vi "Gui_SetupExpert.vi"(8 "error in (no error)":errorcluster, 11 "QMH UI References.Refnum EXPERT":refnum<vi>) -> (0 "error out":errorcluster caption="sortie d'erreur")   [LabVIEW 2024]
doc: "This VI setup the EXPERT parameters.\n\n1. The EXPERT parameters are passed through a Reference as input.\n2. Init the controls with the previous values.\n3. Wait for the user events, and update controls accordingly.\n4. When OK is pushed, the last values of the controls are stored into the address passed by Reference."
uses:
  controls/EXPERT_Inputs.ctl
  controls/DIGIT_5122_Inputs.ctl
  <instrlib>/niScope/Controls/niScope trigger source.ctl
  controls/HSDIO_6541_Inputs.ctl
  <instrlib>/niHSDIO/niHSDIO.llb/niHSDIO_ctl Trigger Source Values (Ring).ctl
  controls/SOFTWARE_Inputs.ctl
  controls/AO_6711_Inputs.ctl
  controls/AWG_5421_Inputs.ctl
  <instrlib>/niFgen/niFgen.llb/niFgen_ctl Trigger Source Values (Ring).ctl
  controls/XML_Inputs.ctl
  controls/AO_6738_Inputs.ctl
panel:
  in  "EXPERT Inputs":T1={"XML Inputs"={"Version Tag Name"="XML_Version", "Version String"="1.0"}, "SOFTWARE Inputs"={"Application Directory"=path "D:/S.O.F.T.S/LABVIEW/PIL", "Software Version"="1.0.0", "Data Path"=path "D:/PIRENEA/DATA", "XML Path"=path "D:/PIRENEA/DATA", "XML File Filter"="*.xml", "XML Saved Path"=path "D:/PIRENEA/DATA/SAVED", "Excit Scripts Path"=path "D:/PIRENEA/EXCIT_SCRIPTS", "Excit Scripts File Filter"="*.txt", "Excit Waveforms Path"=path "D:/PIRENEA/EXCIT_WFMS", "Excit Waveforms File Filter"="*.bin", "Timing Scripts Path"=path "D:/PIRENEA/TIMING_SCRIPTS", "Timing Scripts File Filter"="*.txt", "Timing Waveforms Path"=path "D:/PIRENEA/TIMING_WFMS", "Timing Waveforms File Filter"="*.bin", "Trapping Waveforms Path"=path "D:/PIRENEA/TRAPPING_WFMS", "Trapping Waveforms File Filter"="*.bin"}, "HSDIO 6541 Inputs"={"Resource Name"="HSDIO_6541", "Clock Rate"=1000000.0, "Trigger Source"="PFI0"}, "AWG 5421 Inputs"={"Resource Name"="AWG_5421", "Sample Rate"=10000000.0, "Trigger Type"=2, "Trigger Source"="PFI0", "Waveform Gain"=0.31, "Digital Filter ON"=TRUE}, "DIGIT 5122 Inputs"={"Sample Rate"=10000.0, "Resource Name"="DIGIT_5122", "Channel Name"="0", "Trigger Source"="VAL_EXTERNAL", "Vertical Range"=10.0, "Trigger Level"=3.0}, "AO 6711 Inputs"={"Physical Channels"="AO_6711/ao0:3", "Min Voltage"=-10.0, "Max Voltage"=10.0, "Trigger Source"="/AO_6711/PFI3", "Counter"="AO_6711/ctr0"}, "AO 6738 Inputs"={"Physical Channels"="AO_6738/ao0:3", "Min Voltage"=-10.0, "Max Voltage"=10.0, "Trigger Source"="/AO_6738/PFI2", "Counter"="AO_6738/ctr0"}} {"AO 6738 Inputs"."Max Voltage" min=-10.0 max=10.0; "AO 6738 Inputs"."Min Voltage" min=-10.0 max=10.0; "AWG 5421 Inputs"."Sample Rate" format="%.2p"; "AWG 5421 Inputs"."Trigger Type" items=["None", "Software Edge", "Digital Edge", "Digital Level"]; "AO 6711 Inputs"."Max Voltage" min=-10.0 max=10.0; "AO 6711 Inputs"."Min Voltage" min=-10.0 max=10.0; "HSDIO 6541 Inputs"."Clock Rate" format="%.2p"; "DIGIT 5122 Inputs"."Trigger Level" format="%.2f"; "DIGIT 5122 Inputs"."Vertical Range" format="%.2f"; "DIGIT 5122 Inputs"."Sample Rate" step=65535.0 format="%#_3p"}
  in  "OK":bool
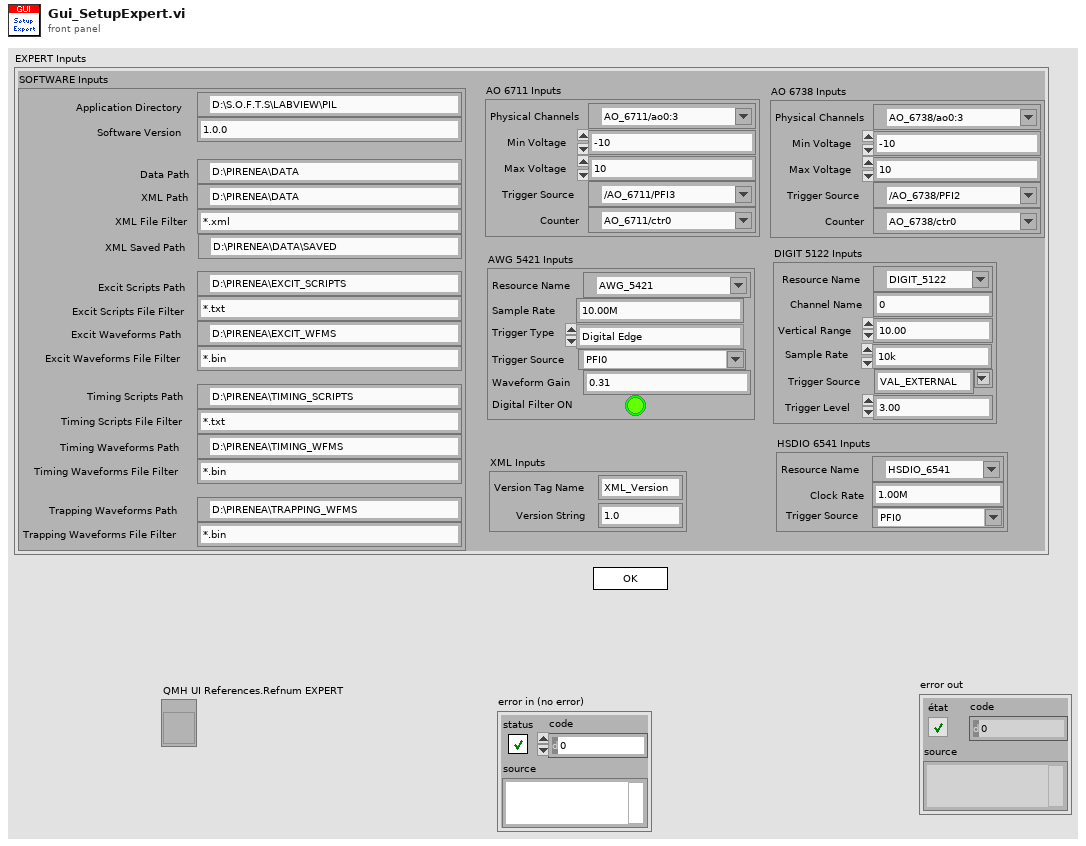
[diagram p1: front panel]
types:
  T1 = typedef "EXPERT_Inputs.ctl" = cluster{"XML Inputs":T2, "SOFTWARE Inputs":T3, "HSDIO 6541 Inputs":T4, "AWG 5421 Inputs":T6, "DIGIT 5122 Inputs":T8, "AO 6711 Inputs":T10, "AO 6738 Inputs":T11}
  T2 = typedef "XML_Inputs.ctl" = cluster{"Version Tag Name":string, "Version String":string}
  T3 = typedef "SOFTWARE_Inputs.ctl" = cluster{"Application Directory":path, "Software Version":string, "Data Path":path, "XML Path":path, "XML File Filter":string, "XML Saved Path":path, "Excit Scripts Path":path, "Excit Scripts File Filter":string, "Excit Waveforms Path":path, "Excit Waveforms File Filter":string, "Timing Scripts Path":path, "Timing Scripts File Filter":string, "Timing Waveforms Path":path, "Timing Waveforms File Filter":string, "Trapping Waveforms Path":path, "Trapping Waveforms File Filter":string}
  T4 = typedef "HSDIO_6541_Inputs.ctl" = cluster{"Resource Name":refnum<k15>, "Clock Rate":dbl, "Trigger Source":T5}
  T5 = typedef "niHSDIO_ctl Trigger Source Values (Ring).ctl" = string
  T6 = typedef "AWG_5421_Inputs.ctl" = cluster{"Resource Name":refnum<k15>, "Sample Rate":dbl, "Trigger Type":u16, "Trigger Source":T7, "Waveform Gain":dbl, "Digital Filter ON":bool}
  T7 = typedef "niFgen_ctl Trigger Source Values (Ring).ctl" = string
  T8 = typedef "DIGIT_5122_Inputs.ctl" = cluster{"Sample Rate":dbl, "Resource Name":refnum<k15>, "Channel Name":string, "Trigger Source":T9, "Vertical Range":dbl, "Trigger Level":dbl}
  T9 = typedef "niScope trigger source.ctl" = string
  T10 = typedef "AO_6711_Inputs.ctl" = cluster{"Physical Channels":tag, "Min Voltage":dbl, "Max Voltage":dbl, "Trigger Source":tag, "Counter":tag}
  T11 = typedef "AO_6738_Inputs.ctl" = cluster{"Physical Channels":tag, "Min Voltage":dbl, "Max Voltage":dbl, "Trigger Source":tag, "Counter":tag}
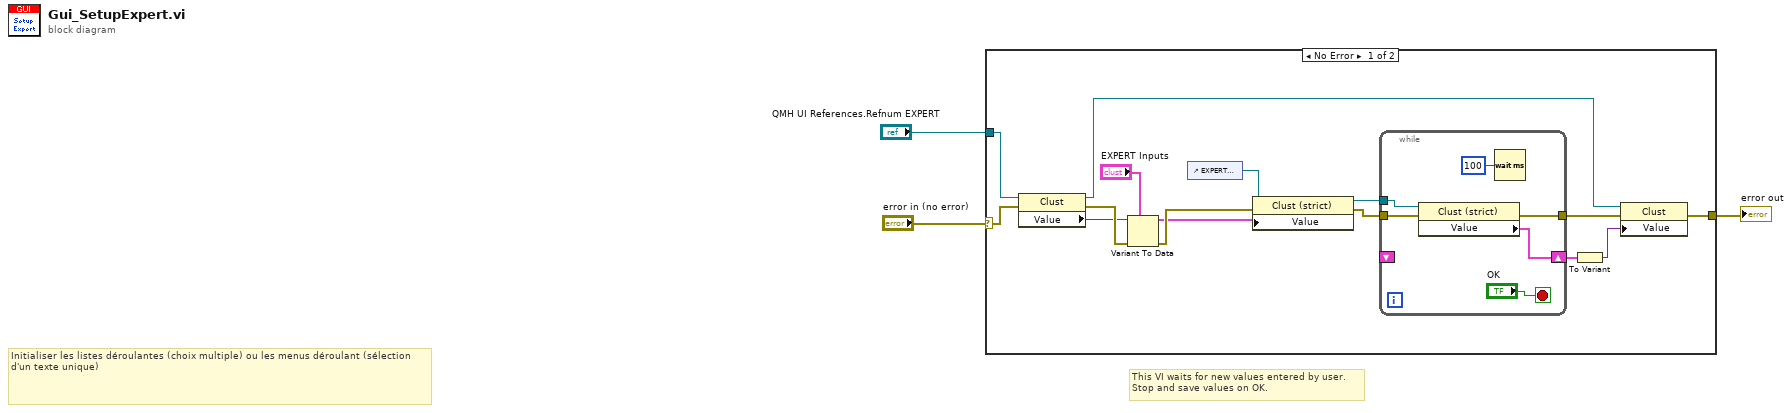
[diagram p0: block diagram]
diagram:
  # "This VI waits for new values entered by user.\nStop and save values on OK."
  # "Initialiser les listes déroulantes (choix multiple) ou les menus déroulant (sélection d'un texte unique)"
  n1 = case shown="No Error" "error in (no error)" {
    selector: "error in (no error)" -> [w11 w25]
    tunnel: [w6 w25] -> w3
    tunnel: "QMH UI References.Refnum EXPERT" -> [w5 _]
    frame No Error {
      n2 = property class="Clust"(reference=w5, error in=w11) -> (reference out=w8:refnum<vi>, error out=w10:errorcluster, "Value"=w9:variant)
      n3 = Variant To Data(error in=w10, type="EXPERT Inputs", Variant=w9) -> (data=w14:T1, error out=w17:errorcluster)
      n4 = control-ref of="EXPERT Inputs"() -> (w4:refnum<vi>)
      n5 = property class="Clust (strict)"(reference=w4, error in=w17, "Value"=w14) -> (reference out=w15:refnum<vi>, error out=w16:errorcluster)
      n6 = while {
        shift-right: [w22] -> w18
        shift-left: _ -> [_]
        tunnel: w16 -> [w21]
        tunnel: w15 -> [w23]
        tunnel: [w20] -> w7
        stop <- "OK" stop-if-true
        n7 = property class="Clust (strict)"(reference=w23, error in=w21) -> (error out=w20:errorcluster, "Value"=w22:T1)  [unwired: 1 out]
        n8 = Wait (ms)(milliseconds to wait=u32 100 ("attente (ms)")) -> ()  [unwired: 1 out]
      }
      n9 = To Variant(anything=w18) -> (Variant=w12:variant)
      n10 = property class="Clust"(reference=w8, error in=w7, "Value"=w12) -> (error out=w6:errorcluster)  [unwired: 1 out]
    }
    frame Error {
    }
  }
  "error out" <- w3
